vi "Test Sync Device.vi"() -> ()   [LabVIEW 2018]
uses:
  Hardware/Synchronization Device/Synchronization Device.lvclass
  C:/Program Files/National Instruments/LabVIEW 2018/vi.lib/ActorFramework/Actor/Actor.lvclass
  Hardware/Synchronization Device Messages/Set Shutter Enable Msg/Set Shutter Enable Msg.lvclass/Set Shutter Enable Msg.ctl
  <vilib>/ActorFramework/Message Enqueuer/Message Enqueuer.lvclass/Message Enqueuer.ctl
  Hardware/Synchronization Device Messages/Set Interval Msg/Set Interval Msg.lvclass/Set Interval Msg.ctl
  <vilib>/ActorFramework/Message Enqueuer/Enqueue.vi
  Hardware/Synchronization Device Messages/Set Shutter Enable Msg/Set Shutter Enable Msg.lvclass
  C:/Program Files/National Instruments/LabVIEW 2018/vi.lib/ActorFramework/Message/Message.lvclass
  Hardware/Synchronization Device Messages/Set Interval Msg/Set Interval Msg.lvclass
  <vilib>/ActorFramework/Stop Msg/Stop Msg.lvclass
  Resources/GLOBAL/GLOBAL Time-critical.vi
  <vilib>/ActorFramework/Message Priority Queue/Priority Enqueue.vi
  <vilib>/ActorFramework/Actor/Actor.lvclass
panel:
  in  "Shutter Enable":bool[](array[boolean])
  out "Current Frame":i32
  in  "Shutter Lines":string[](array[string])=["Dev1/port1/line0", "Dev1/port1/line1", "Dev1/port1/line2", "Dev1/port1/line3"]
  in  "ALEX":bool=TRUE
  in  "Camera Sync Channel":string="Dev1/port2/line7"
  in  "Interval (ms)":dbl=200.0
  in  "stop":bool
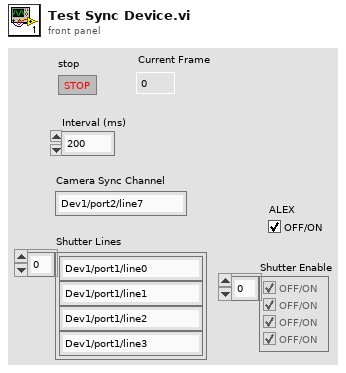
[diagram p1: front panel]
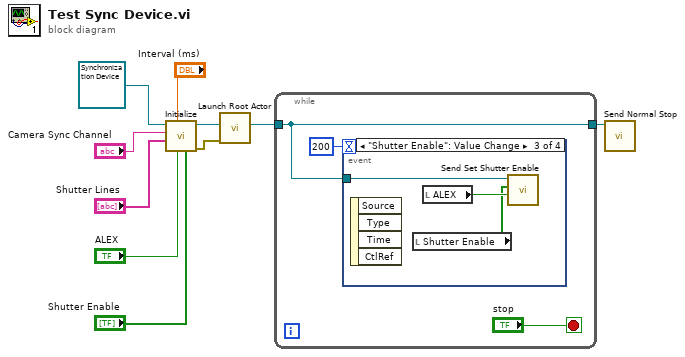
[diagram p0: block diagram]
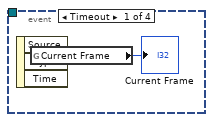
[diagram p2: hidden frame]
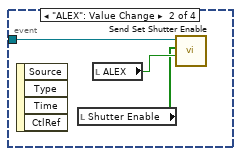
[diagram p3: hidden frame]
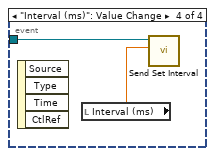
[diagram p4: hidden frame]
diagram:
  n1 = call "Initialize.vi"("Shutter Enable"="Shutter Enable", "ALEX"="ALEX", "Interval (ms)"="Interval (ms)", "Shutter Lines"="Shutter Lines", "Sync Line"="Camera Sync Channel", "Synchronization Device in"=refnum<class "Synchronization Device.lvclass"> refnum ("Synchronization Device.lvlib:Synchronization Device.lvclass")) -> ("error out"=w5:errorcluster, "Synchronization Device out"=w7:refnum<class "Synchronization Device.lvclass">)  [unwired: 4 in]
  n2 = call <vilib>:"Launch Root Actor.vi"("error in (no error)"=w5, "Actor"=w7) -> ("Actor's Enqueuer"=w10:refnum<class "Message Enqueuer.lvclass">)  [unwired: 8 in, 1 out]
  n3 = while {
    tunnel: w10 -> [w12]
    tunnel: [w12] -> w9
    stop <- "stop" stop-if-true
    n4 = event shown="[2] \"Shutter Enable\": Value Change" {
      selector: _ -> [_ _ _ _]
      dyn-events: _ -> [_ _ _ _]
      timeout: 200 -> [_ _ _ _]
      tunnel: w12 -> [_ w17 w20 w21]
      event Timeout {
        n5 = event-data() -> ()  [unwired: 1 in, 3 out]
        n6 = global read "GLOBAL Time-critical.vi" "Current Frame"() -> (→"Current Frame":i32)
      }
      event "ALEX": Value Change {
        n7 = event-data() -> ()  [unwired: 1 in, 4 out]
        n8 = local read "Shutter Enable"() -> (w15:bool[])
        n9 = local read "ALEX"() -> (w16:bool)
        n10 = call "Send Set Shutter Enable.vi"("ALEX?"=w16, "Shutter Enable"=w15, "Message Enqueuer"=w17) -> ()  [unwired: 7 in, 2 out]
      }
      event "Shutter Enable": Value Change {
        n11 = event-data() -> ()  [unwired: 1 in, 4 out]
        n12 = local read "Shutter Enable"() -> (w18:bool[])
        n13 = local read "ALEX"() -> (w19:bool)
        n14 = call "Send Set Shutter Enable.vi"("ALEX?"=w19, "Shutter Enable"=w18, "Message Enqueuer"=w20) -> ()  [unwired: 7 in, 2 out]
      }
      event "Interval (ms)": Value Change {
        n15 = event-data() -> ()  [unwired: 1 in, 4 out]
        n16 = local read "Interval (ms)"() -> (w22:dbl)
        n17 = call "Send Set Interval.vi"("Interval (ms)"=w22, "Message Enqueuer"=w21) -> ()  [unwired: 8 in, 2 out]
      }
    }
  }
  n18 = call <vilib>:"Send Normal Stop.vi"("Message Enqueuer"=w9) -> ()  [unwired: 10 in, 1 out]
